vi "Platform 송신.vi"() -> (0 "Platform Protocol Error":errorcluster)   [LabVIEW 2016]
uses:
  <vilib>/Platform/TimedLoop/XDataNode/timing_clust.ctl
  <vilib>/Platform/TimedLoop/XDataNode/nitl_modes.ctl
  <vilib>/Platform/TimedLoop/XDataNode/wakeup.ctl
  <vilib>/Platform/TimedLoop/XDataNode/XDataNode.xnode
  <vilib>/Platform/TimedLoop/XDataNode/XDNodeRunTimeDep.lvlib
panel:
  in  "Platform error in":errorcluster
  in  "Platform Baud rate":u32(ring)=115200 items=["Auto Connect"=0, "300"=300, "600"=600, "1200"=1200, "2400"=2400, "4800"=4800, "9600"=9600, "19200"=19200, "38400"=38400, "57600"=57600, "115200"=115200]
  out "hex string":string
  in  "stop?":bool
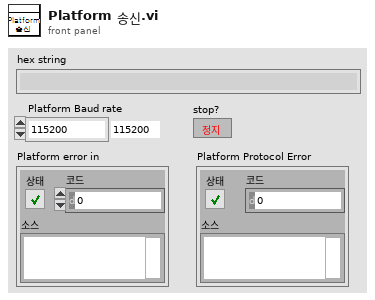
[diagram p1: front panel]
types:
  T1 = typedef "XDNodeRunTimeDep.lvlib/timing_clust.ctl" = cluster{"Expected End [f-1]":u64, "Actual End [f-1]":u64, "Finished Late? [f-1]":bool, "Expected End [i-1]":u64, "Actual End [i-1]":u64, "Finished Late? [i-1]":bool, "Expected Start [i]":u64, "Actual Start [i]":u64, "Expected Start [f]":u64, "Actual Start [f]":u64, "Source Name":string, "Structure Name":string, "Period":i64, "Deadline":i64, "Offset":i64, "Start":i64, "Priority":i32, "Timeout":i32, "Mode":T2, "Wakeup Reason":T3, "Error":errorcluster, "Source Type":string, "Secondary Source Type":string, "Global End Time":u64, "Global Start Time":u64, "Frame Duration":u64, "Iteration Duration":u64, "Assigned CPU":i32, "I/O Scan Engine Mode":u32}
  T2 = typedef "XDNodeRunTimeDep.lvlib/nitl_modes.ctl" = enum32{"No Change", "Process missed periods, maintain original phase", "Discard missed periods, maintain original phase", "Process missed periods, ignore original phase", "Discard missed periods, ignore original phase"}
  T3 = typedef "XDNodeRunTimeDep.lvlib/wakeup.ctl" = enum32{"Normal", "Aborted", "Asynchronous wakeup", "Timing source error", "Timed loop error", "Timeout"}
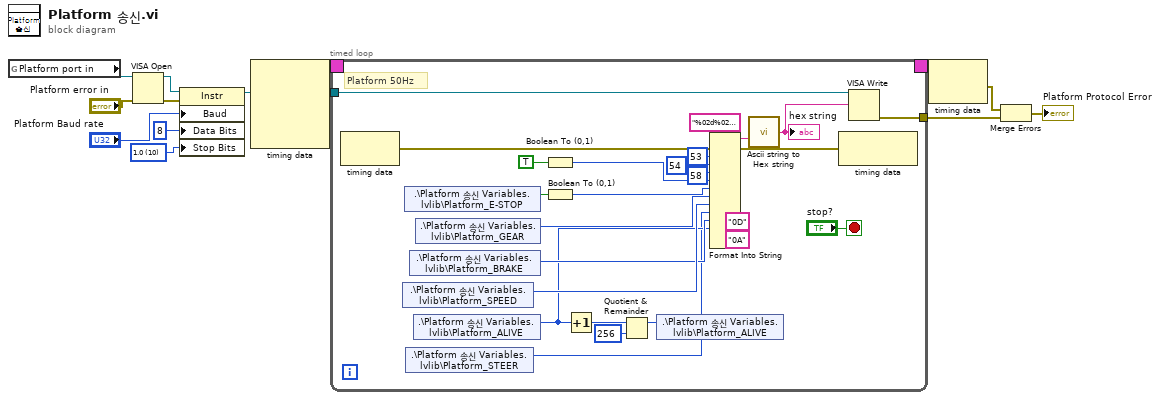
[diagram p0: block diagram]
diagram:
  w2 = u16 10 items=["1.0"=10, "1.5"=15, "2.0"=20] ("Serial Settings:Stop Bits")
  n1 = global read "[GV]_PLATFORM Port NUM.vi" "Platform port in"() -> (w1:refnum<visa-resource-name>)
  n2 = VISA Open(error in (no error)="Platform error in", VISA resource name=w1) -> (VISA resource name=w5:refnum<visa-resource-name>, error out=w7:errorcluster)  [unwired: 3 in]
  n3 = property class="Instr"(reference=w5, error in=w7, "Baud"="Platform Baud rate", "Data Bits"=u16 8 ("Serial Settings:Data Bits"), "Stop Bits"=w2) -> (reference out=w3:refnum<visa-resource-name>)  [unwired: 1 out]
  n4 = node-c288() -> (w13:T1)  [unwired: 4 in]
  n5 = timed-loop {
    timing: w13 -> [_]
    timing-out: [_] -> w12
    tunnel: [w33] -> w10
    tunnel: w3 -> [w27]
    stop <- "stop?" stop-if-true
    # "Platform 50Hz"
    n6 = node-c288() -> (w35:errorcluster)  [unwired: 1 in]
    n7 = shared-variable ".\\Platform 송신 Variables.lvlib\\Platform_SPEED"() -> (w20:u16)  [unwired: 1 in, 1 out]
    n8 = shared-variable ".\\Platform 송신 Variables.lvlib\\Platform_E-STOP"() -> (w32:bool)  [unwired: 1 in, 1 out]
    n9 = shared-variable ".\\Platform 송신 Variables.lvlib\\Platform_STEER"() -> (w15:i16)  [unwired: 1 in, 1 out]
    n10 = shared-variable ".\\Platform 송신 Variables.lvlib\\Platform_BRAKE"() -> (w19:u16)  [unwired: 1 in, 1 out]
    n11 = shared-variable ".\\Platform 송신 Variables.lvlib\\Platform_ALIVE"() -> (w16:u16)  [unwired: 1 in, 1 out]
    n12 = shared-variable ".\\Platform 송신 Variables.lvlib\\Platform_GEAR"() -> (w21:u16)  [unwired: 1 in, 1 out]
    n13 = Boolean To (0,1)(Boolean=TRUE ("Platform_A or M")) -> (0, 1=w23:i16)
    n14 = Boolean To (0,1)(Boolean=w32) -> (0, 1=w22:i16)
    n15 = Increment(x=w16) -> (x+1=w37:u16)
    n16 = Quotient & Remainder(x=w37, y=u16 256) -> (x-y*floor(x/y)=w31:u16)  [unwired: 1 out]
    n17 = shared-variable ".\\Platform 송신 Variables.lvlib\\Platform_ALIVE"(w31) -> ()  [unwired: 1 in, 1 out]
    n18 = Format Into String(format string="%02d%02d%02d%02x%02x%02x%04x%04x%02x%02x%02s%02s" ("포맷 문자열"), error in=w35, u16 53 ("S"), u16 54 ("T"), u16 58 ("X"), w23, w22, w21, w20, w15, w19, w16, "0D" ("ETX0"), "0A" ("ETX1")) -> (resulting string=w29:string, error out=w34:errorcluster)  [unwired: 1 in]
    n19 = call "Ascii string to Hex string.vi"("ASCII String"=w29) -> ("HEX String"=w28:string)
    "hex string" <- w28
    n20 = node-c288(w34) -> ()  [unwired: 1 out]
    n21 = VISA Write(VISA resource name=w27, write buffer=w28) -> (error out=w33:errorcluster)  [unwired: 1 in, 2 out]
  }
  n22 = node-c288(w12) -> (w11:errorcluster)
  n23 = Merge Errors(w11, w10) -> (→"Platform Protocol Error":errorcluster)
